vi "Auto Elevator Mode.vi"(0 "Elevator Command":T3={"Command"=enum."Idle", "Manual Motor Out"=0.0, "Manual Eject Piston"=FALSE, "Mode"=enum."Manual", "Override Limits"=FALSE, "Manual Stabilizer"=FALSE, "Manual Finger"=FALSE, "Store Trashcan?"=FALSE, "Hold Low?"=FALSE, "Idle Mode"=enum."Load Can", "HP Load"=FALSE, "Unstick"=FALSE, "Raw Height Set"=0.0, "Force Store"=FALSE}, 2 "reinitialize? (F)":bool, 5 "Current Position":dbl, 7 "High IR":bool, 9 "Object In?":bool, 11 "Finger Height":dbl) -> (4 "Auto Elevator Indicators":T1, 6 "output":dbl, 8 "Finger Out":bool, 10 "Stabilizer Out":bool, 14 "Finger at bottom":bool, 15 "Eject Out":bool)   [LabVIEW 2014]
uses:
  Elevator Control Command.ctl
  Elevator Command.ctl
  Common Code/Elevator Mode.ctl
  Common Code/Elevator Idle Mode.ctl
  Common Code/Auto Elevator Indicators.ctl
  Common Code/Elevator State.ctl
  Elevator Sensors.ctl
  Common Code/Utilities/TimeManager.vi
  Common Code/Change Detect.vi
  Common Code/Change Detect Boolean.vi
  Robot Global Data.vi
  <vilib>/addons/control/pid/pid.llb/PID (DBL).vi
  <vilib>/addons/control/pid/NI_PID_pid.lvlib
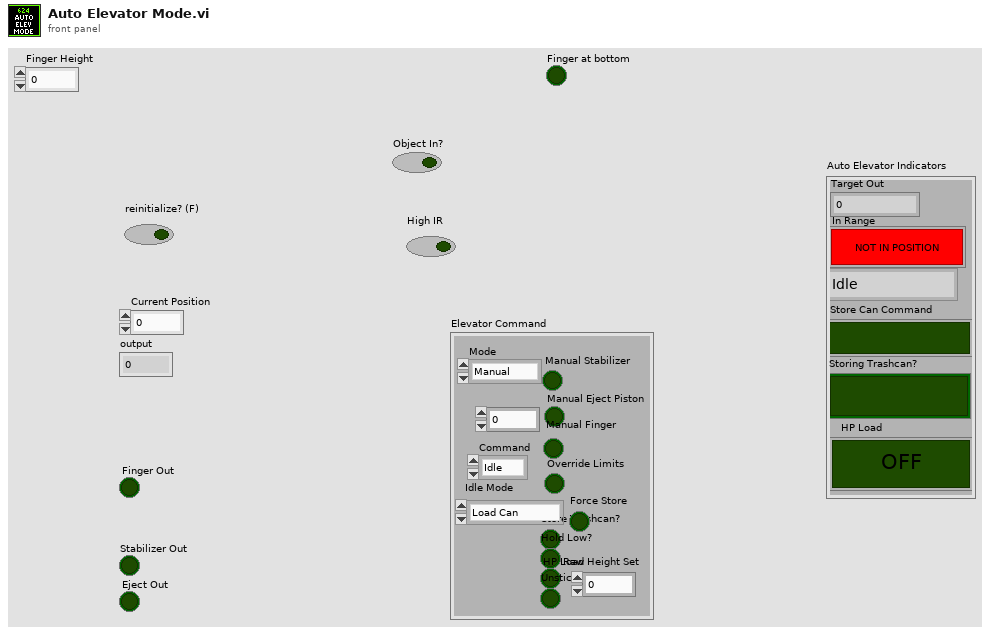
[diagram p1: front panel]
types:
  T1 = typedef "Auto Elevator Indicators.ctl" = cluster{"Target Out":dbl, "Storing Trashcan?":bool, "State":T2, "In Range":bool, "Store Can Command":bool, "HP Load":bool}
  T2 = typedef "Elevator State.ctl" = enum16{"Idle", "Goto Load Position", "Wait for Load", "Load Drop", "Load Lift", "Drop Stack", "Goto Eject Position", "Eject ", "Raise Trashcan", "Open Stabilizer", "Untip Drop", "Untip Wait", "Untip Lift", "Abort Load", "HP Load Wait", "HP Load Drop", "HP Load Lift", "HP Load Abort", "Close Stabilizer", "HP Load Unfinish", "HP Load Score", "HP Load Finish", "HP Goto Finish Down", "HP Goto Finish Up", "Full"}
  T3 = typedef "Elevator Control Command.ctl" = cluster{"Command":T4, "Manual Motor Out":dbl, "Manual Eject Piston":bool, "Mode":T5, "Override Limits":bool, "Manual Stabilizer":bool, "Manual Finger":bool, "Store Trashcan?":bool, "Hold Low?":bool, "Idle Mode":T6, "HP Load":bool, "Unstick":bool, "Raw Height Set":dbl, "Force Store":bool}
  T4 = typedef "Elevator Command.ctl" = enum16{"Idle", "Load 1", "Load 2", "Load 3", "Drop Stack", "Eject Stack", "Untip Trashcan", "Load Trashcan", "HP Load", "HP Score"}
  T5 = typedef "Elevator Mode.ctl" = enum16{"Manual", "Safe", "Auto"}
  T6 = typedef "Elevator Idle Mode.ctl" = enum16{"Load 1", "Load 2", "Load 3", "Load Can", "Untip Can", "Step Load", "Drop Stack", "Raw Height"}
  T7 = typedef "Elevator Status.ctl" = cluster{"Height":dbl, "Enc Value":dbl, "Limit Override":bool, "Mode":T5, "High IR":bool, "Motor Out":dbl, "Ping Detect":bool, "Auto Elevator Indicators":T1, "Master Current":dbl, "Slave Current":dbl, "High Current":bool, "Current Tripped":bool, "Top Limit":bool, "Bottom Limit":bool, "Eject Piston":bool, "Stabilizer":bool, "Finger":bool, "Finger Height":dbl, "Finger Raw":dbl, "Finger at Bottom":bool}
  T8 = typedef "Elevator Sensors.ctl" = cluster{"Object In?":bool, "Elevator in Position?":bool, "Current Position":dbl, "Abort Load":bool, "Finger Height":dbl, "Finger at bottom?":bool, "Rollers Out of Way?":bool, "High IR":bool}
  T9 = typedef "Dashboard Control Data.ctl" = cluster{"Cam Exposure":dbl, "Go to angle":dbl, "Steer PID Gains":cluster{"proportional gain (Kc)":dbl, "integral time (Ti, min)":dbl, "derivative time (Td, min)":dbl}, "Steer PID output Range":cluster{"output high":dbl, "output low":dbl}, "Pressure m \nValue":dbl, "Pressure b \nValue":dbl, "Roller Command Cluster ":T10, "Elevator":T11, "Encoder Control":T13, "Auton Settings":cluster{"Drive Dist Window Size":dbl}, "Drivetrain Settings":T14, "Lance":T15}
  T10 = typedef "Roller Control.ctl" = cluster{"Intake Speed":dbl, "Turn In Speed":dbl, "Unload Speed":dbl, "Turn Out Speed":dbl, "Ping Align Tolerance":dbl, "Tote Range Threshold":dbl, "Right Pot 0":dbl, "Pot Threshold":dbl, "Left Pot 0":dbl, "Right Pot Scale":dbl, "Left Pot Scale":dbl, "Min Elevator Height":dbl, "Eject Time":dbl, "Eject US Threshold":dbl, "Anti-Twitch Time":u32, "Ping Caring Threshold":dbl, "Pot Diff Threshold":dbl, "Pinch Sustain":u32, "Absorb Give Up Threshold":dbl, "Untip In Threshold":dbl, "Untip Grab Range":dbl, "Ultrasonic Hold Time":u32, "Landscape Absorb Time":u32, "Pot Use Wait Time":u32, "Can Turn Stop Range":dbl, "HP Load Speed":dbl, "Stick Multiplier":dbl}
  T11 = typedef "Elevator DB Control.ctl" = cluster{"PID Output Range":cluster{"output high":dbl, "output low":dbl}, "PID gains":cluster{"proportional gain (Kc)":dbl, "integral time (Ti, min)":dbl, "derivative time (Td, min)":dbl}, "Height Tolerance":sgl, " Encoder Constant":dbl, "Eject Time":sgl, "Zeroing Speed":sgl, "Presets":T12, "Ping Detect Threshold":sgl, "Trashcan Detect Threshold":sgl, "Zero Filter Time":dbl, "Stabilizer Open Time":dbl, "Zero Creep Speed":dbl, "Max Current":dbl, "Current Trip Time":dbl, "Abort Pitch":dbl, "Finger m":dbl, "Finger b":dbl, "Finger max ":dbl, "Finger Stabilizer":dbl, "Finger Store":dbl, "Finger Stop Store":dbl, "Stabilizer Close Time":dbl, "Finger min":dbl, "Unstick gain":dbl}
  T12 = typedef "Elevator Presets.ctl" = cluster{"Pickup 2 w/ Tote":sgl, "Pickup 2 w/ Trashcan":sgl, "Pickup 3 w/ Tote":sgl, "Pickup 3 w/ Trashcan":sgl, "Bottom":sgl, "Pickup 1 w/ Tote":sgl, "Pickup Trashcan":sgl, "Pickup 1 w/ Trashcan":sgl, "Eject":sgl, "Hold Low":sgl, "Step add height":sgl, "Untip Lift":dbl, "Drop Stack":dbl, "HP Load Hold":dbl, "HP Load Drop":dbl, "HP Load Hold Can":dbl, "Store can max":dbl, "HP Drag Score":dbl, "HP Drag Finish":dbl, "Finger trashcan avoid":dbl, "Full":dbl}
  T13 = typedef "Encoder Control.ctl" = cluster{"Left Tick Constant":dbl, "Right Tick Constant":dbl, "Center Tick Constant":dbl, "Reset?":bool, "Y Dist":cluster{"PID gains":cluster{"proportional gain (Kc)":dbl, "integral time (Ti, min)":dbl, "derivative time (Td, min)":dbl}}, "X Dist":cluster{"PID gains":cluster{"proportional gain (Kc)":dbl, "integral time (Ti, min)":dbl, "derivative time (Td, min)":dbl}}, "Y Stop Thresh":dbl, "Y Stop Speed":dbl, "X Stop Thresh":dbl, "X Stop Speed":dbl}
  T14 = typedef "Drivetrain Settings.ctl" = cluster{"Gyro Tolerance":sgl, "Strafe Correct max steer":sgl, "Strafe Timer Wait":sgl, "Throttle Ramp (ms)":sgl, "Strafe Ramp (ms)":sgl, "Angular rate compensation":bool, "Throttle to Rate Scale":sgl, "Rate compensation gain":sgl, "Creep Steer":sgl, "Creep Throttle":sgl}
  T15 = typedef "Pike DB Controls.ctl" = cluster{"Down Speed":dbl, "Up Speed":dbl, "Max Down Time":dbl, "Max Up Time":dbl, "Current Limit":dbl}
  T16 = typedef "Roller Indicators.ctl" = cluster{"Rollers Closed?":bool, "Roller Mode":T17, "Auto Roller State":T18, "Tote Inside?":bool, "Intake State":T19, "Left Ping Dist":sgl, "Right Ping Dist":sgl, "Potentiometer Cluster":T20, "PING Decision":T19, "Left Arm Closed?":bool, "Portrait?":bool, "Right Arm Closed?":bool, "Left Out":sgl, "Right Out":sgl, "Left Current":sgl, "Right Current":sgl, "Tote Load Complete?":bool, "Untip Complete?":bool, "Untip State":T21, "Roller Safety Open":bool}
  T17 = typedef "Roller Mode Enum.ctl" = enum16{"Manual", "Safe", "Auto"}
  T18 = typedef "Auto Roller Commands.ctl" = enum16{"Drag Tote", "Grab Tote", "Idle", "Eject Tote", "Untip Can", "Grab Can"}
  T19 = typedef "Inner Roller States.ctl" = enum16{"Turn Tote Portrait", "Acquire Tote", "Absorb Tote", "Turn Tote Right", "Turn Tote Left", "Acquire Can", "Absorb Can", "Turn Can", "Hold Tote"}
  T20 = typedef "Pot Data.ctl" = cluster{"Left Pot Zero":sgl, "Right Pot Zero":sgl, "Left Potentiometer":sgl, "Right Potentiometer":sgl, "Left Pot Non Zero":sgl, "Right Pot Non Zero":sgl}
  T21 = typedef "Untip Can States.ctl" = enum16{"Release Can", "Catch Can", "Idle"}
  T22 = typedef "IMU Data.ctl" = cluster{"Pitch":sgl, "Roll":sgl, "Yaw":sgl, "Data Valid?":bool, "Temp":sgl, "MOVING":bool, "NAVX_CAL_STATUS":T23, "NAVX_OP_STATUS":T24, "YAW_STABLE":bool, "Accel X":sgl, "Accel Y":sgl, "Accel Z":sgl, "Accel Magnitude":sgl, "Pitch Rate":sgl, "Roll Rate":sgl, "Yaw Rate":sgl, "NavX Opened?":bool}
  T23 = typedef "navX-MXP IMU.lvlib/navX NAVX_CAL_STATUS.ctl" = u8
  T24 = typedef "navX-MXP IMU.lvlib/navX NAVX_OP_STATUS.ctl" = u8
  T25 = cluster{"proportional gain (Kc)":dbl, "integral time (Ti, min)":dbl, "derivative time (Td, min)":dbl}
  T26 = typedef "Elevator Actuators.ctl" = cluster{"Ejector Piston":bool, "Finger":bool, "Stabilizer":bool, "Position Out":dbl}
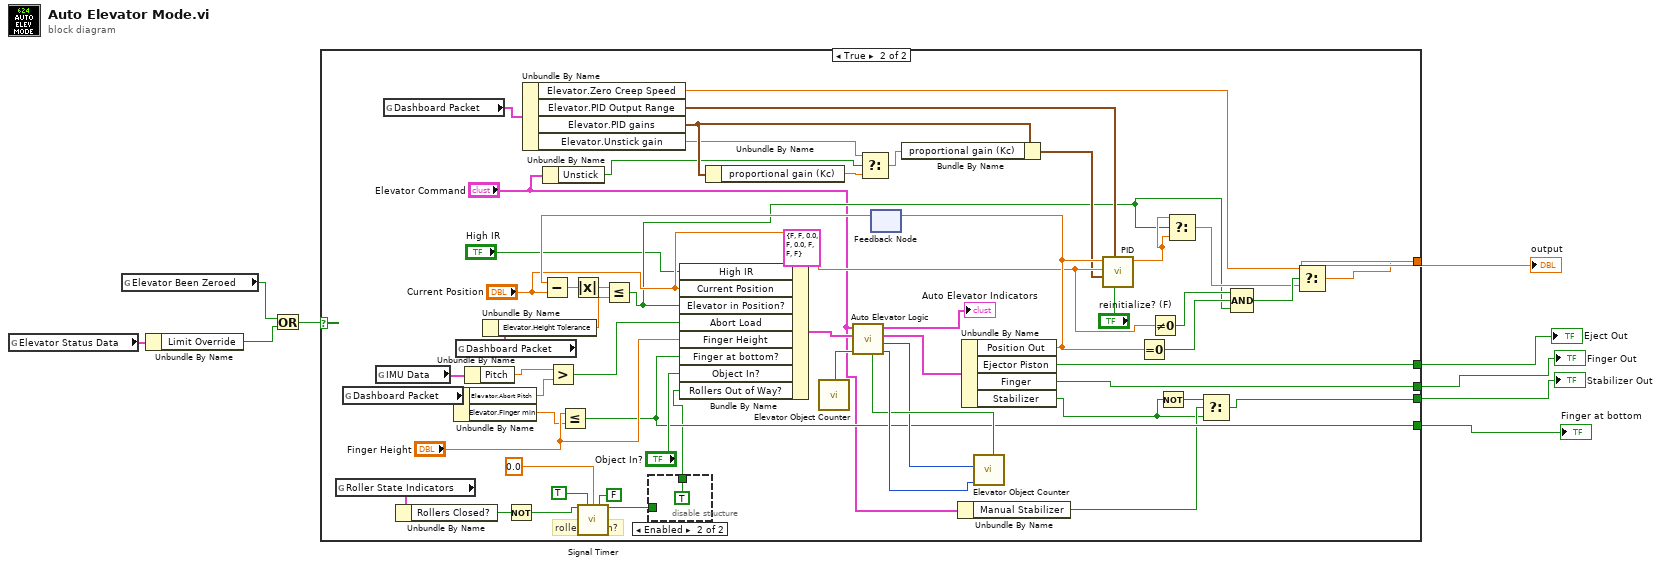
[diagram p0: block diagram]
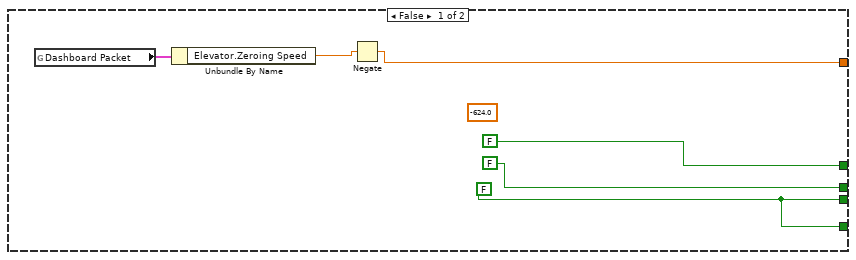
[diagram p2: hidden frame]
diagram:
  n1 = global read "Robot Global Data.vi" "Elevator Status Data"() -> (w5:T7)
  n2 = global read "Robot Global Data.vi" "Elevator Been Zeroed"() -> (w4:bool)
  n3 = Unbundle By Name(w5) -> ("Limit Override"=w3:bool)
  n4 = Or(x=w4, y=w3) -> (x .or. y?=w2:bool)
  n5 = case shown="True" w2 {
    tunnel: [w11 w16] -> w9
    tunnel: [FALSE ("Ejector Piston") w59] -> w8
    tunnel: [FALSE ("Finger") w58] -> w7
    tunnel: [w10 w23] -> w6
    tunnel: [w10 w38] -> w1
    frame False {
      (unwired) -624.0 ("Position Out")
      w10 = FALSE ("Stabilizer")
      n6 = global read "Robot Global Data.vi" "Dashboard Packet"() -> (w13:T9)
      n7 = Unbundle By Name(w13) -> ("Elevator.Zeroing Speed"=w12:sgl)
      n8 = Negate(x=w12) -> (-x=w11:sgl)
    }
    frame True {
      # "rollers open?"
      n9 = global read "Robot Global Data.vi" "Roller State Indicators"() -> (w30:T16)
      n10 = global read "Robot Global Data.vi" "Dashboard Packet"() -> (w49:T9)
      n11 = global read "Robot Global Data.vi" "IMU Data"() -> (w51:T22)
      n12 = global read "Robot Global Data.vi" "Dashboard Packet"() -> (w65:T9)
      n13 = Unbundle By Name(w30) -> ("Rollers Closed?"=w29:bool)
      n14 = Unbundle By Name(w49) -> ("Elevator.Abort Pitch"=w48:dbl, "Elevator.Finger min"=w39:dbl)
      n15 = global read "Robot Global Data.vi" "Dashboard Packet"() -> (w57:T9)
      n16 = Unbundle By Name(w51) -> ("Pitch"=w50:sgl)
      n17 = Unbundle By Name(w57) -> ("Elevator.Height Tolerance"=w68:sgl)
      n18 = Not(x=w29) -> (.not. x?=w28:bool)
      n19 = Unbundle By Name(w65) -> ("Elevator.Zero Creep Speed"=w53:dbl, "Elevator.PID Output Range"=w64:cluster{"output high":dbl, "output low":dbl}, "Elevator.PID gains"=w37:T25, "Elevator.Unstick gain"=w34:dbl)
      n20 = Unbundle By Name("Elevator Command") -> ("Unstick"=w32:bool)
      n21 = Greater?(x=w50, y=w48) -> (0:w47:bool)
      n22 = Less Or Equal?(x="Finger Height", y=w39) -> (x <= y?=w38:bool)
      n23 = call "Signal Timer.vi"("Input"=w28, "Edge"=TRUE, "Interval"=0.0, "Pull"=FALSE) -> ("Filtered Output"=w20:bool)  [unwired: 11 in]
      n24 = disable-structure shown="Enabled" {
        disable-tunnel: w20 -> [w73 _]
        disable-tunnel: [w73 TRUE ("Filtered Output")] -> w19
        frame Disabled {
        }
        frame Enabled {
        }
      }
      n25 = Unbundle By Name(w37) -> ("proportional gain (Kc)"=w35:dbl)
      n26 = call "Elevator Object Counter.vi"() -> ("Have Trashcan"=w63:bool)  [unwired: 10 in, 1 out]
      n27 = Select(t=w34, s=w32, f=w35) -> (s? t:f=w33:dbl)
      n28 = feedback #1() -> (w69:dbl)  [unwired: 1 in]
      n29 = Subtract(x=w69, y="Current Position") -> (x-y=w71:dbl)
      n30 = Absolute Value(x=w71) -> (abs(x)=w72:dbl)
      n31 = Less Or Equal?(x=w72, y=w68) -> (x <= y?=w31:bool)
      n32 = Bundle By Name(cluster=T8 {"Object In?"=FALSE, "Elevator in Position?"=FALSE, "Current Position"=0.0, "Abort Load"=FALSE, "Finger Height"=0.0, "Finger at bottom?"=FALSE, "Rollers Out of Way?"=FALSE, "High IR"=FALSE} ("Elevator Sensors In"), "High IR"="High IR", "Current Position"="Current Position", "Elevator in Position?"=w31, "Abort Load"=w47, "Finger Height"="Finger Height", "Finger at bottom?"=w38, "Object In?"="Object In?", "Rollers Out of Way?"=w19) -> (w66:T8)
      n33 = call "Auto Elevator Logic.vi"("Has Trashcan?"=w63, "Elevator Sensors In"=w66, "Command"="Elevator Command") -> ("Trashcan Delta"=w62:i32, "Tote Delta"=w41:i16, "Elevator Actuators Out"=w70:T26, "Auto Elevator Indicators"=→"Auto Elevator Indicators":T1, "Clear Stack Count"=w60:bool)  [unwired: 4 in]
      n34 = Bundle By Name(cluster=w37, "proportional gain (Kc)"=w33) -> (w36:T25)
      n35 = Unbundle By Name("Elevator Command") -> ("Manual Stabilizer"=w24:bool)
      n36 = Unbundle By Name(w70) -> ("Position Out"=w55:dbl, "Ejector Piston"=w59:bool, "Finger"=w58:bool, "Stabilizer"=w21:bool)
      n37 = feedback-in #1(w55) -> ()
      n38 = call "Elevator Object Counter.vi"("Clear Stack?"=w60, "Trashcan Delta"=w62, "Tote Delta"=w41) -> ()  [unwired: 7 in, 2 out]
      n39 = call-poly <vilib>:"PID.vi"("reinitialize? (F)"="reinitialize? (F)", "output range"=w64, "PID gains"=w36, "process variable"="Current Position", "setpoint"=w55) -> ("output"=w45:dbl)  [unwired: 5 in, 1 out]
      n40 = Equal To 0?(x=w55) -> (x = 0?=w43:bool)
      n41 = Not Equal To 0?(x="Current Position") -> (x != 0?=w44:bool)
      n42 = Not(x=w21) -> (.not. x?=w22:bool)
      n43 = Select(t=w45, s=w31, f=w45) -> (s? t:f=w46:dbl)
      n44 = Select(t=w22, s=w24, f=w21) -> (s? t:f=w23:bool)
      n45 = Compound Arithmetic op=AND(w44, w43, w31) -> (w52:bool)
      n46 = Select(t=w53, s=w52, f=w46) -> (s? t:f=w16:dbl)
    }
  }
  "output" <- w9
  "Eject Out" <- w8
  "Finger Out" <- w7
  "Stabilizer Out" <- w6
  "Finger at bottom" <- w1
